vi "LPS22HH CONF REG2.vi"(8 "error in":errorcluster, 11 "instrument handle":refnum<k15>) -> (0 "error out":errorcluster, 3 "instrument handle out":refnum<k15>)   [LabVIEW 2020, in "LPS22Demo.lvlib"]
uses:
  <instrlib>/niDigital/niDigital.llb/niDigital Write Source Waveform (Broadcast U32).vi
  <instrlib>/niDigital/niDigital.llb/niDigital Burst Pattern (Burst Only).vi
  LPS22Demo.lvlib
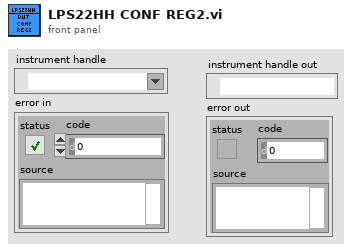
[diagram p1: front panel]
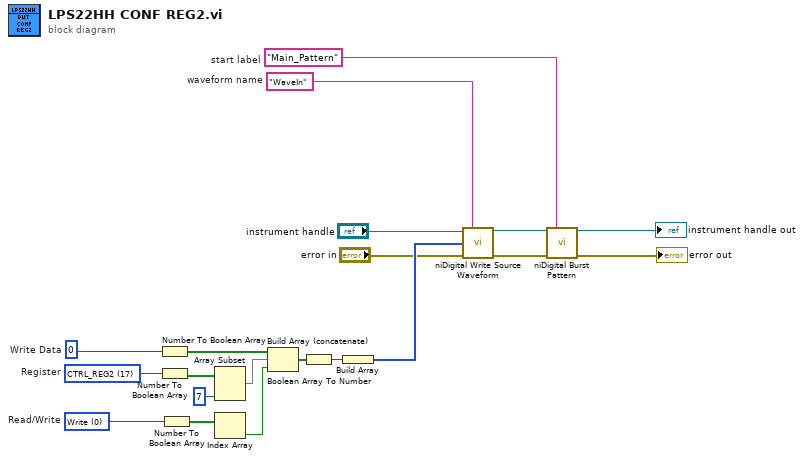
[diagram p0: block diagram]
diagram:
  w3 = "Main_Pattern"  # start label
  w11 = i16 0 items=["Write", "Read"]  # Read/Write
  w13 = u16 17 items=["INTERRUPT_CFG"=11, "THS_P_L"=12, "THS_P_H"=13, "IF_CTRL"=14, "WHO_AM_I"=15, "CTRL_REG1"=16, "CTRL_REG2"=17, "CTRL_REG3"=18, "FIFO_CTRL"=19, "FIFO_WTM"=20, "RPDS_L"=24, "RPDS_H"=25, "INT_SOURCE"=36, "FIFO_STATUS1"=37, "FIFO_STATUS2"=38, "STATUS"=39, "PRESSURE_OUT_XL"=40, "PRESSURE_OUT_L"=41, "PRESSURE_OUT_H"=42, "TEMP_OUT_L"=43, "TEMP_OUT_H"=44, "FIFO_DATA_OUT_PRESS_XL"=120, "FIFO_DATA_OUT_PRESS_L"=121, "FIFO_DATA_OUT_PRESS_H"=122, "FIFO_DATA_OUT_TEMP_L"=123, "FIFO_DATA_OUT_TEMP_H"=124]  # Register
  w17 = i8 0  # Write Data
  w4 = "WaveIn"  # waveform name
  n1 = Number To Boolean Array(number=w17) -> (Boolean array=w18:bool[])
  n2 = Number To Boolean Array(number=w13) -> (Boolean array=w14:bool[])
  n3 = Number To Boolean Array(number=w11) -> (Boolean array=w12:bool[])
  n4 = Array Subset(array=w14, length=7) -> (w15:bool[])  [unwired: 1 in]
  n5 = Index Array(array=w12) -> (element=w16:bool)  [unwired: 1 in]
  n6 = Build Array (concatenate)(w18, w15, w16) -> (w19:bool[])
  n7 = Boolean Array To Number(Boolean array=w19) -> (number=w20:u32)
  n8 = Build Array(w20) -> (w9:u32[])
  n9 = call-poly <instrlib>:"niDigital Write Source Waveform.vi"("instrument handle"="instrument handle", "waveform name"=w4, "waveform data"=w9, "error in"="error in") -> ("instrument handle out"=w7:refnum<k15>, "error out"=w8:errorcluster)  [unwired: 10 in]
  n10 = call-poly <instrlib>:"niDigital Burst Pattern.vi"("instrument handle"=w7, "start label"=w3, "error in"=w8) -> ("instrument handle out"=→"instrument handle out":refnum<k15>, "error out"=→"error out":errorcluster)  [unwired: 11 in]
